vi "function A.vi"(8 "stop":bool, 9 "volume":dbl, 10 "frequency 2":dbl, 11 "frequency 1":dbl) -> (1 "AccelerationZ":i16, 2 "AccelerationY":i16, 3 "AccelerationX":i16)   [LabVIEW 2016]
uses:
  <vilib>/FPGAPlugInAG/myRIO-1900/niLvFpga_Open_myRIO-1900.vi
  <vilib>/rvi/interface/common/dynamic/niFpgaDynamicAddResources.vi
  <vilib>/Utility/error.llb/Error Cluster From Error Code.vi
  <vilib>/rvi/errors/niLvFpgaAdjustHostInterfaceError.vi
  <vilib>/FPGAPlugInAG/Dynamic/niLvFpga_Close_Dynamic.vi
  <vilib>/rvi/interface/nirviOpenFPGA/nirviOpenFPGA.xnode
  FPGA Bitfiles/Musicbox_FPGATarget_soundctrl_6-HSKECpU5c.lvbitx
  sound_ctrl.vi
  <vilib>/rvi/interface/nirviReadWriteControl/nirviReadWriteControl.xnode
  <vilib>/rvi/interface/nirviCloseFPGA/nirviCloseFPGA.xnode
  NiFpgaLv.dll
  <vilib>/rvi/interface/Simulation/niFpgaSimulationCallBeginRW.vi
panel:
  out "error out":errorcluster
  out "Frequency Indicator":dbl
  out "Volume Indicator":dbl
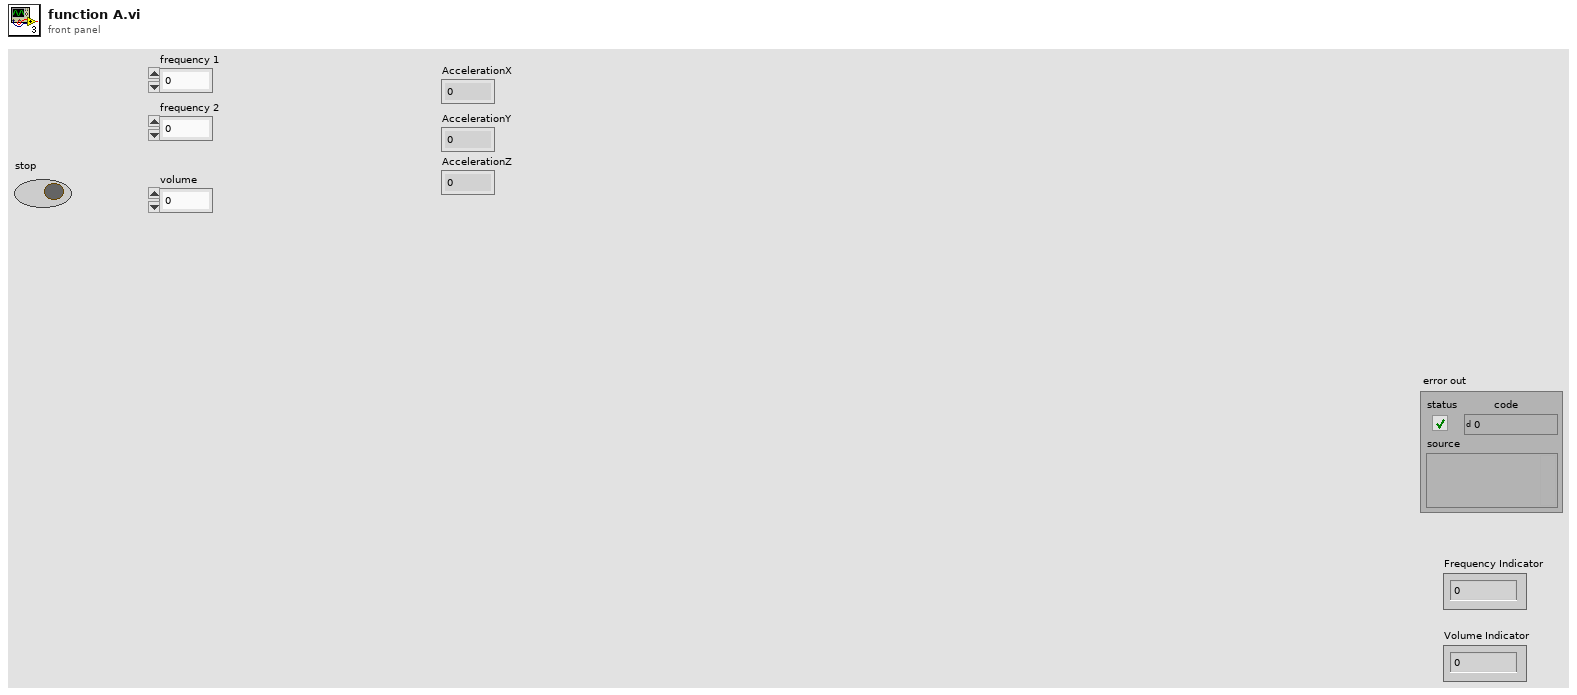
[diagram p1: front panel]
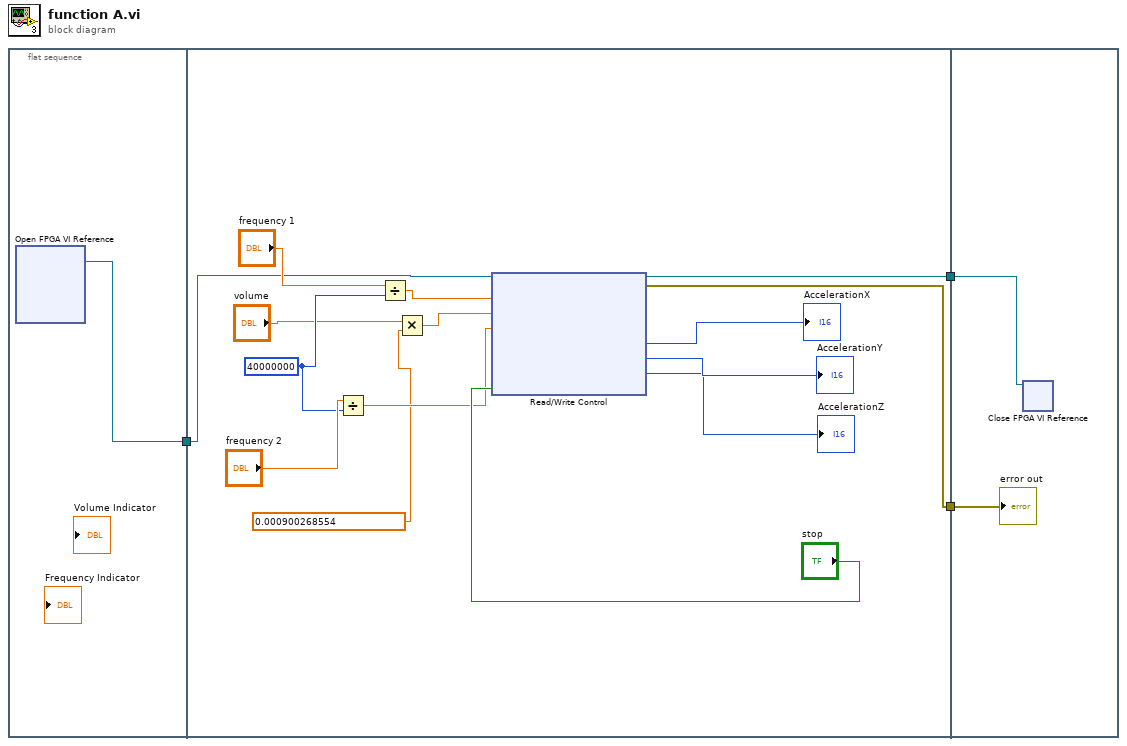
[diagram p0: block diagram]
diagram:
  n1 = flat-sequence {
    tunnel: [w4] -> w3
    tunnel: w3 -> [w6]
    tunnel: [w7] -> w2
    tunnel: [w5] -> w1
    tunnel: w2 -> [w21]
    tunnel: w1 -> [w20]
    frame #0 {
      n2 = xnode "Open FPGA VI Reference"() -> ("FPGA VI Reference Out"=w4:refnum<k20>)  [unwired: 2 in, 1 out]
    }
    frame #1 {
      w9 = 40000000
      n3 = Divide(x="frequency 2", y=w9) -> (x/y=w17:dbl)
      n4 = Divide(x="frequency 1", y=w9) -> (x/y=w18:dbl)
      n5 = Multiply(x="volume", y=0.000900268554) -> (x*y=w16:dbl)
      n6 = xnode ("Read/Write Control")("FPGA VI Reference In"=w6, "frequency (periods/tick)"=w18, "Volume"=w16, "frequency (periods/tick) 2"=w17, "stop"="stop") -> ("FPGA VI Reference Out"=w7:refnum<k20>, "error out"=w5:errorcluster, "AccelerationX"=→"AccelerationX":i16, "AccelerationY"=→"AccelerationY":i16, "AccelerationZ"=→"AccelerationZ":i16)  [unwired: 1 in]
    }
    frame #2 {
      n7 = xnode "Close FPGA VI Reference"("FPGA VI Reference In"=w21) -> ()  [unwired: 1 in, 1 out]
      "error out" <- w20
    }
  }
